vi "ai_continuous_full.vi"() -> ()   [LabVIEW 2020]
uses:
  <vilib>/Analysis/baseanly.llb/Mean (DBL).vi
  <vilib>/Analysis/NI_AALBase.lvlib
panel:
  out "数组":dbl[](array[numeric]) format="%.5f"
  out "Rounds":i32
  out "error out":errorcluster caption="错误输出"
  out "AiFifoResidual":i32
  in  "Stop":bool
  out "波形图":sgl[][](graph)
  in  "PointsToRead":u32=2000
  in  "SamplePeriod(ns)":u32=2000
  in  "ChanSel":bool[](array[boolean])=[TRUE, TRUE, TRUE, FALSE, FALSE, FALSE, FALSE, FALSE, FALSE, FALSE, FALSE, FALSE, FALSE, FALSE, FALSE, FALSE, FALSE, FALSE, FALSE, FALSE, FALSE, FALSE, FALSE, FALSE]
  # "500k"
  # "2000"
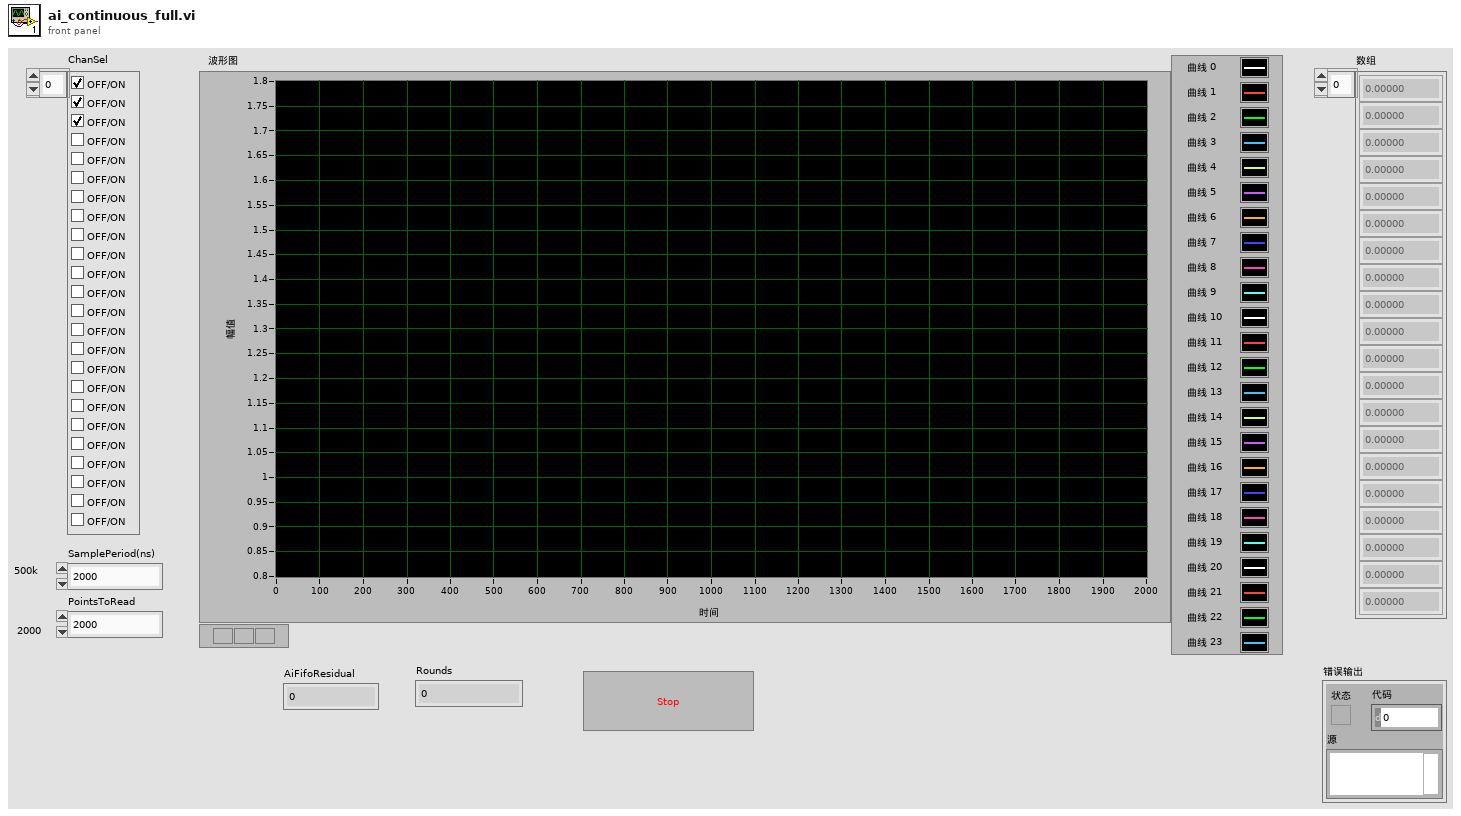
[diagram p1: front panel]
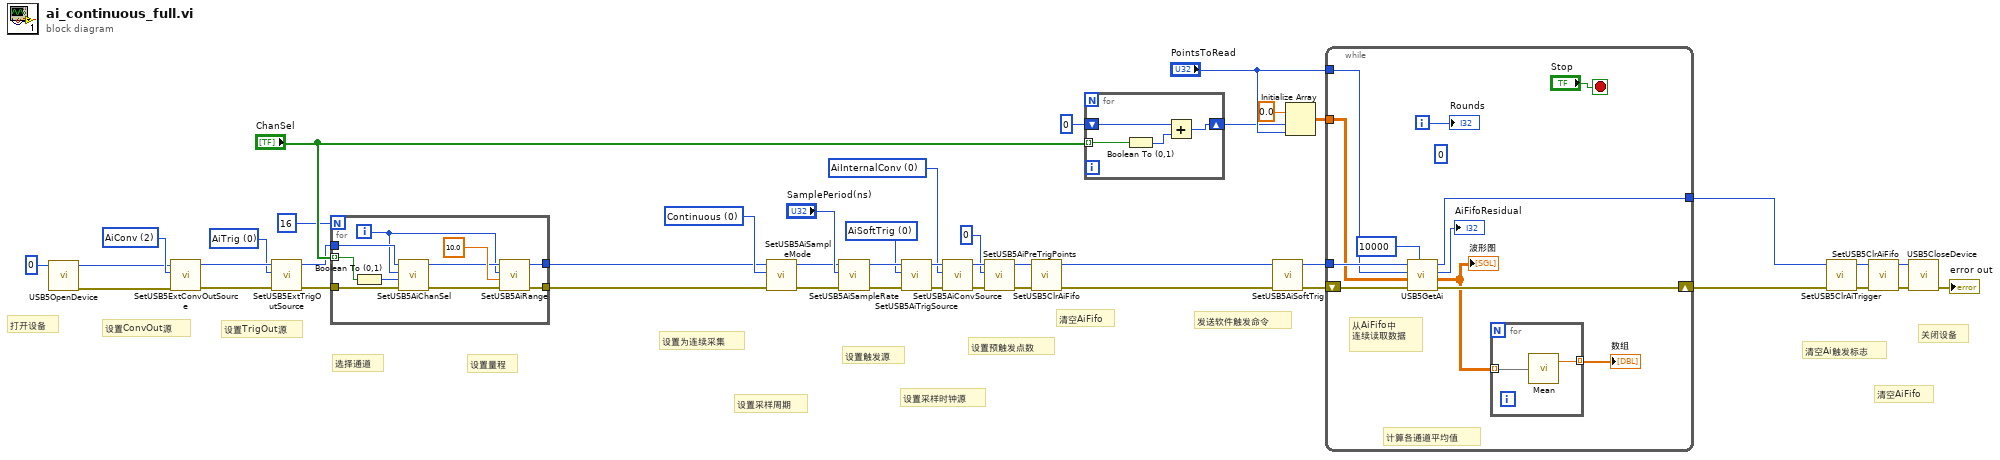
[diagram p0: block diagram]
diagram:
  w6 = u8 0 items=["AiInternalConv"=0, "ConvIn"=1, "DiConv"=3, "DoConv"=4, "Ao0Conv"=5, "Ao1Conv"=6, "Ao2Conv"=7, "Ao3Conv"=8] ("AiConvSource")
  w7 = u8 0 items=["AiSoftTrig"=0, "ExtTrigIn"=1, "Din0RisingEdge"=2, "Din1RisingEdge"=3, "Din2RisingEdge"=4, "Din3RisingEdge"=5, "WithDiTrig"=7, "WithDoTrig"=8, "WithAo0Trig"=9, "WithAo1Trig"=10, "WithAo2Trig"=11, "WithAo3Trig"=12, "GlobalSoftTrig"=255] ("AiTrigSource")
  w8 = u8 0 items=["AiTrig", "DiTrig", "DoTrig", "Ao0Trig", "Ao1Trig", "Ao2Trig", "Ao3Trig"] ("Source")
  w9 = u8 2 items=["AiConv"=2, "DiConv"=3, "DoConv"=4, "Ao0Conv"=5, "Ao1Conv"=6, "Ao2Conv"=7, "Ao3Conv"=8] ("Source")
  w42 = u8 0 items=["Continuous", "OneShot"] ("AiSampleMode")
  # "设置量程"
  # "关闭设备"
  # "清空AiFifo"
  # "清空Ai触发标志"
  # "发送软件触发命令"
  # "清空AiFifo"
  # "设置预触发点数"
  # "设置采样时钟源"
  # "设置触发源"
  # "设置采样周期"
  # "设置为连续采集"
  # "选择通道"
  # "设置TrigOut源"
  # "设置ConvOut源"
  # "打开设备"
  n1 = call "USB5OpenDevice.vi"("DevIndex"=0) -> ("error out"=w1:errorcluster, "DevIndex Out"=w2:i32)  [unwired: 9 in]
  n2 = call "SetUSB5ExtConvOutSource.vi"("错误输入（无错误）"=w1, "Source"=w9, "DevIndex"=w2) -> ("错误输出"=w12:errorcluster, "DevIndex Out"=w13:i32)  [unwired: 7 in]
  n3 = call "SetUSB5ExtTrigOutSource.vi"("错误输入（无错误）"=w12, "Source"=w8, "DevIndex"=w13) -> ("错误输出"=w16:errorcluster, "DevIndex Out"=w17:i32)  [unwired: 7 in]
  n4 = for {
    N: 16 -> [_]
    tunnel: w17 -> [w54]
    tunnel: w16 -> [w53]
    tunnel: "ChanSel" -> [w51] mode=indexing
    tunnel: [w46] -> w5
    tunnel: [w45] -> w4
    i -> [w47]
    n5 = Boolean To (0,1)(Boolean=w51) -> (0, 1=w52:i16)
    n6 = call "SetUSB5AiChanSel.vi"("错误输入（无错误）"=w53, "Sel"=w52, "Chan"=w47, "DevIndex"=w54) -> ("错误输出"=w48:errorcluster, "DevIndex Out"=w49:i32)  [unwired: 6 in]
    n7 = call "SetUSB5AiRange.vi"("错误输入（无错误）"=w48, "AiRange"=sgl 10.0, "Chan"=w47, "DevIndex"=w49) -> ("错误输出"=w45:errorcluster, "DevIndex Out"=w46:i32)  [unwired: 6 in]
  }
  n8 = call "SetUSB5AiSampleMode.vi"("错误输入（无错误）"=w4, "AiSampleMode"=w42, "DevIndex"=w5) -> ("错误输出"=w10:errorcluster, "DevIndex Out"=w11:i32)  [unwired: 7 in]
  n9 = call "SetUSB5AiSampleRate.vi"("错误输入（无错误）"=w10, "SamplePeriod(ns)"="SamplePeriod(ns)", "DevIndex"=w11) -> ("错误输出"=w40:errorcluster, "DevIndex Out"=w41:i32)  [unwired: 7 in]
  n10 = call "SetUSB5AiTrigSource.vi"("错误输入（无错误）"=w40, "AiTrigSource"=w7, "DevIndex"=w41) -> ("错误输出"=w38:errorcluster, "DevIndex Out"=w39:i32)  [unwired: 7 in]
  n11 = call "SetUSB5AiConvSource.vi"("错误输入（无错误）"=w38, "AiConvSource"=w6, "DevIndex"=w39) -> ("错误输出"=w36:errorcluster, "DevIndex Out"=w37:i32)  [unwired: 7 in]
  n12 = call "SetUSB5AiPreTrigPoints.vi"("错误输入（无错误）"=w36, "AiPreTrigPoints"=u32 0, "DevIndex"=w37) -> ("错误输出"=w33:errorcluster, "DevIndex Out"=w34:i32)  [unwired: 7 in]
  n13 = call "SetUSB5ClrAiFifo.vi"("错误输入（无错误）"=w33, "DevIndex"=w34) -> ("错误输出"=w14:errorcluster, "DevIndex Out"=w15:i32)  [unwired: 8 in]
  n14 = for {
    tunnel: "ChanSel" -> [w58] mode=indexing
    shift-right: [w55] -> w22
    shift-left: i16 0 -> [w56]
    n15 = Boolean To (0,1)(Boolean=w58) -> (0, 1=w57:i16)
    n16 = Add(x=w56, y=w57) -> (x+y=w55:i16)
  }
  n17 = call "SetUSB5AiSoftTrig.vi"("错误输入（无错误）"=w14, "DevIndex"=w15) -> ("错误输出"=w31:errorcluster, "DevIndex Out"=w32:i32)  [unwired: 8 in]
  n18 = Initialize Array(sgl 0.0 ("元素"), w22, "PointsToRead") -> (w27:sgl[][])
  n19 = while {
    tunnel: w32 -> [w70]
    tunnel: "PointsToRead" -> [w68]
    tunnel: w27 -> [w62]
    tunnel: [w66] -> w19
    shift-right: [w65] -> w18
    shift-left: w31 -> [w69]
    i -> [w63]
    stop <- "Stop" stop-if-true
    (unwired) 0 ("禁用的索引 (列)")
    # "计算各通道平均值"
    # "从AiFifo中\n连续读取数据"
    n20 = call "USB5GetAi.vi"("TimeOut"=10000, "错误输入（无错误）"=w69, "Ai"=w62, "Points"=w68, "DevIndex"=w70) -> ("错误输出"=w65:errorcluster, "Ai Out"=w60:sgl[][], "AiFifoUsed"=→"AiFifoResidual":i32, "DevIndex Out"=w66:i32)  [unwired: 3 in]
    "波形图" <- w60
    n21 = for {
      tunnel: w60 -> [w72] mode=indexing
      tunnel: [w71] -> w59 mode=indexing
      n22 = call-poly <vilib>:"Mean.vi"("X"=w72) -> ("mean"=w71:dbl)  [unwired: 1 out]
    }
    "数组" <- w59
    "Rounds" <- w63
  }
  n23 = call "SetUSB5ClrAiTrigger.vi"("错误输入（无错误）"=w18, "DevIndex"=w19) -> ("错误输出"=w20:errorcluster, "DevIndex Out"=w21:i32)  [unwired: 8 in]
  n24 = call "SetUSB5ClrAiFifo.vi"("错误输入（无错误）"=w20, "DevIndex"=w21) -> ("错误输出"=w26:errorcluster, "DevIndex Out"=w25:i32)  [unwired: 8 in]
  n25 = call "USB5CloseDevice.vi"("错误输入（无错误）"=w26, "DevIndex"=w25) -> ("error out"=→"error out":errorcluster)  [unwired: 8 in, 1 out]
